vi "Global Setup.vi"(8 "error in (no error)":errorcluster, 11 "Global Fixture Test Double in":refnum<class "Global Fixture Test Double.lvclass">) -> (0 "error out":errorcluster)   [LabVIEW 2020, in "Global Fixture Test Double.lvclass"]
uses:
  Global Fixture Test Double.lvclass
  Global Variable.vi
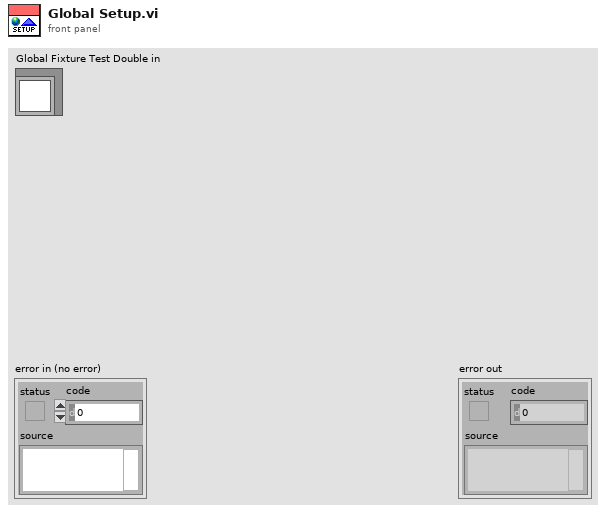
[diagram p1: front panel]
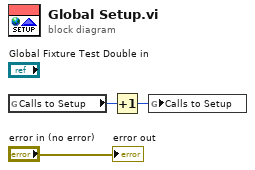
[diagram p0: block diagram]
diagram:
  n1 = global read "Global Variable.vi" "Calls to Setup"() -> (w2:i32)
  n2 = Increment(x=w2) -> (x+1=w1:i32)
  n3 = global write "Global Variable.vi" "Calls to Setup"(w1) -> ()
  "error out" <- "error in (no error)"
